vi "Read or create tokens on LabVIEW INI.vi"(8 "error in":errorcluster, 10 "New Value":string, 11 "Token":string) -> (0 "error out":errorcluster, 2 "found?":bool, 3 "Value":string)   [LabVIEW 2021]
doc: "Reads token from LabVIEW INI file specified by \"key\"\nIf token does not exist, it creates it and tries to read it back."
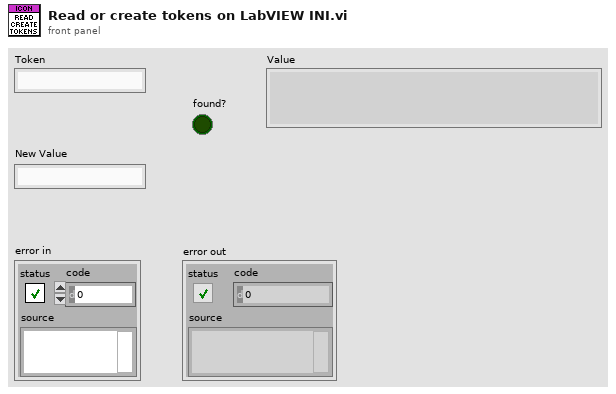
[diagram p1: front panel]
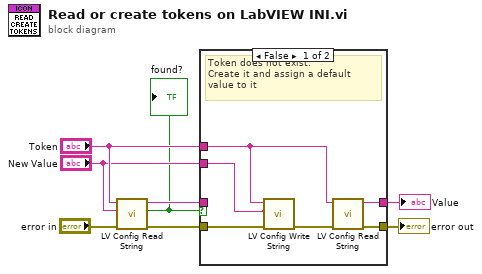
[diagram p0: block diagram]
diagram:
  n1 = call <resource>:"LV Config Read String.vi"("error in"="error in", "default value"="New Value", "key"="Token") -> ("error out"=w7:errorcluster, "found?"=w2:bool, "value"=w4:string)  [unwired: 2 in]
  "found?" <- w2
  n2 = case shown="False" w2 {
    tunnel: w7 -> [w14 w16]
    tunnel: "Token" -> [w12 _]
    tunnel: "New Value" -> [w9 _]
    tunnel: [w11 w16] -> w5
    tunnel: [w10 w15] -> w1
    tunnel: w4 -> [_ w15]
    frame False {
      # "Token does not exist. \nCreate it and assign a default value to it"
      n3 = call <resource>:"LV Config Write String.vi"("error in (no error)"=w14, "value"=w9, "key"=w12) -> ("error out"=w13:errorcluster)  [unwired: 4 in]
      n4 = call <resource>:"LV Config Read String.vi"("error in"=w13, "key"=w12) -> ("error out"=w11:errorcluster, "value"=w10:string)  [unwired: 3 in, 1 out]
    }
    frame True {
      # "Token exists"
    }
  }
  "error out" <- w5
  "Value" <- w1
